vi "Set TagIDs.vi"(8 "error in (no error)":errorcluster, 10 "Folder Info":T2, 11 "Station Actor in":refnum<class "Station Actor.lvclass">) -> (0 "error out":errorcluster, 3 "Station Actor out":refnum<class "Station Actor.lvclass">)   [LabVIEW 2019, in "Station Actor.lvlib" / "Station Actor.lvclass"]
uses:
  Station Actor.lvclass
  <vilib>/OPCUA/controls/OPC UA Server Refnum.ctl
  Station Actor.lvclass/Station Actor.ctl
  <vilib>/OPCUA/controls/Data Type.ctl
  <vilib>/OPCUA/NI OPC UA Server.lvlib
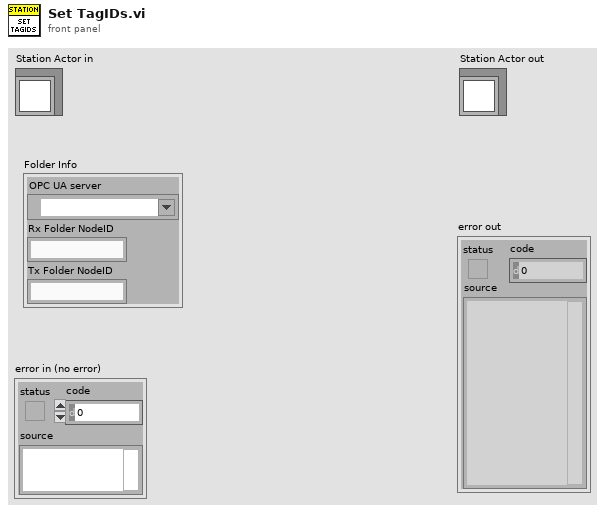
[diagram p1: front panel]
types:
  T1 = typedef "OPC UA Server Refnum.ctl" = refnum<k21>
  T2 = cluster{"OPC UA server":T1, "Rx Folder NodeID":string, "Tx Folder NodeID":string}
  T3 = typedef "Data Type.ctl" = u16
  T4 = cluster{"name":string, "data type":T3, "access level":u16, "description":string}
  T5 = typedef "NodeId.ctl" = string
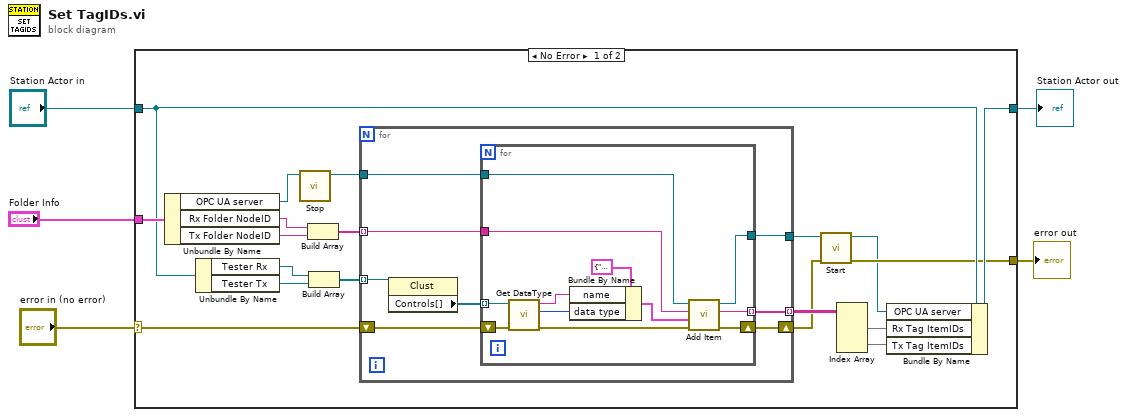
[diagram p0: block diagram]
diagram:
  n1 = case shown="No Error" "error in (no error)" {
    selector: "error in (no error)" -> [w8 w46]
    tunnel: [w7 w46] -> w4
    tunnel: [w10 w45] -> w2
    tunnel: "Station Actor in" -> [w11 w45]
    tunnel: "Folder Info" -> [w22 _]
    frame No Error {
      n2 = Unbundle By Name(w22) -> ("OPC UA server"=w19:T1, "Rx Folder NodeID"=w21:string, "Tx Folder NodeID"=w20:string)
      n3 = Unbundle By Name(w11) -> ("Tester Rx"=w24:refnum<vi>, "Tester Tx"=w23:refnum<vi>)
      n4 = call <vilib>:"Stop.vi"("OPC UA server refnum in"=w19) -> ("OPC UA server refnum out"=w18:T1)  [unwired: 9 in, 1 out]
      n5 = Build Array(w21, w20) -> (w17:string[])
      n6 = Build Array(w24, w23) -> (w16:refnum<vi>[])
      n7 = for {
        tunnel: w17 -> [w30] mode=indexing
        tunnel: [w29] -> w12 mode=indexing
        shift-right: [w31] -> w9
        shift-left: w8 -> [w32]
        tunnel: w18 -> [w27]
        tunnel: [w26] -> w13
        tunnel: w16 -> [w25] mode=indexing
        n8 = property class="Clust"(reference=w25) -> ("Controls[]"=w28:refnum<vi>[])  [unwired: 1 in, 2 out]
        n9 = for {
          tunnel: w30 -> [w44]
          shift-right: [w43] -> w31
          shift-left: w32 -> [w38]
          tunnel: [w42] -> w29 mode=indexing
          tunnel: w28 -> [w39] mode=indexing
          tunnel: w27 -> [w34]
          tunnel: [w33] -> w26
          n10 = call "Get DataType.vi"("error in (no error)"=w38, "reference"=w39) -> ("error out"=w36:errorcluster, "data type"=w35:T3, "Name"=w37:string)  [unwired: 7 in]
          n11 = Bundle By Name(cluster=T4 {"name"="", "data type"=1, "access level"=3, "description"=""} ("item"), "name"=w37, "data type"=w35) -> (w40:T4)
          n12 = call <vilib>:"Add Item.vi"("error in (no error)"=w36, "item"=w40, "parent folder node ID"=w44, "OPC UA server refnum in"=w34) -> ("error out"=w43:errorcluster, "item node ID"=w42:T5, "OPC UA server refnum out"=w33:T1)  [unwired: 3 in, 1 out]
        }
      }
      n13 = call <vilib>:"Start.vi"("error in (no error)"=w9, "OPC UA server refnum in"=w13) -> ("error out"=w7:errorcluster, "OPC UA server refnum out"=w6:T1)  [unwired: 7 in, 1 out]
      n14 = Index Array(array=w12) -> (element #1=w14:T5[], element #2=w15:T5[])  [unwired: 4 in]
      n15 = Bundle By Name(cluster=w11, "OPC UA server"=w6, "Rx Tag ItemIDs"=w14, "Tx Tag ItemIDs"=w15) -> (w10:refnum<class "Station Actor.lvclass">)
    }
    frame Error {
    }
  }
  "error out" <- w4
  "Station Actor out" <- w2
